vi "Periodic Tasks.vi"(8 "error in":errorcluster) -> ()   [LabVIEW 2014]
doc: "This VI runs in parallel to other tasks. It can contain as many user-defined periodic loops as you need. These can carry out PID or other sorts of timed response."
uses:
  <vilib>/Rock Robotics/WPI/Joystick/WPI_JoystickGetSetRefNum.vi
  <vilib>/Rock Robotics/WPI/RobotDrive/WPI_RobotDriveGetSetRefNum.vi
  <vilib>/Rock Robotics/WPI/RobotDrive/WPI_RobotDriveMotorSelectorEnum.ctl
  <vilib>/Rock Robotics/SystemInterfaces/NetworkCommunication/NetComm_UsageReport_ResourceType.ctl
  <vilib>/addons/control/pid/NI_PID_pid.lvlib
  <vilib>/addons/control/pid/pid.llb/PID (DBL).vi
  Robot Global Data.vi
  robotics/labview/nav6/roborio/labview/Nav6Library/Nav6.lvlib
panel:
  out "Motor Values":dbl[](array[numeric])
  in  "Gyro Angle":dbl
  in  "error in (no error)":errorcluster
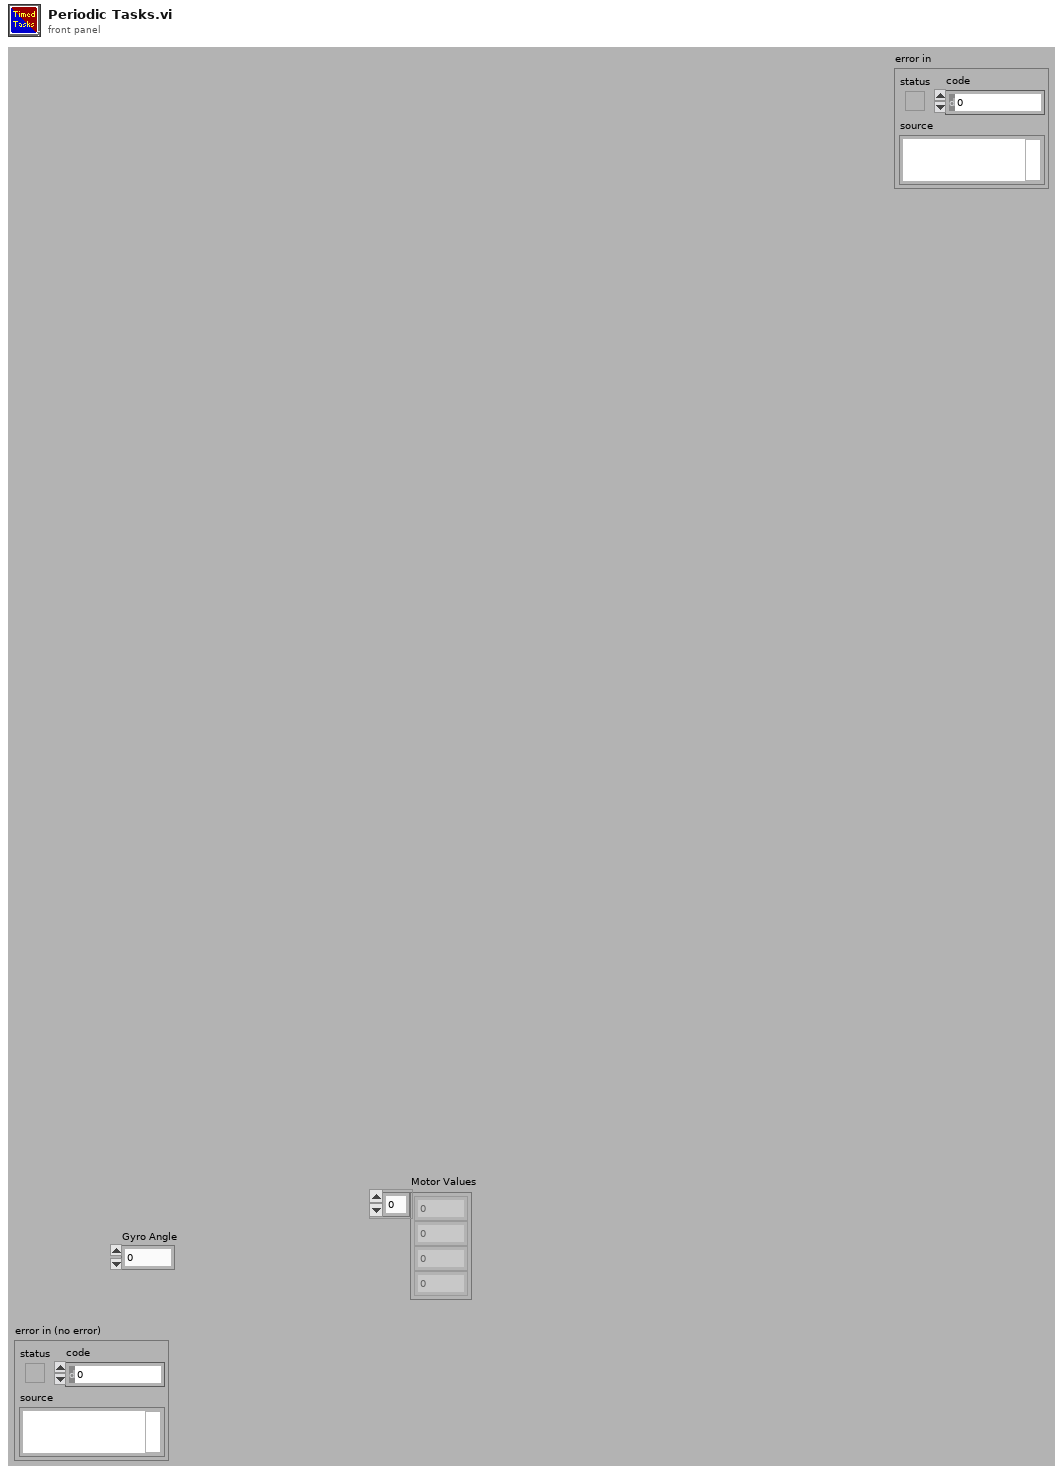
[diagram p1: front panel]
types:
  T1 = typedef "NetComm_UsageReport_ResourceType.ctl" = enum8{"Controller", "Module", "Language", "CANPlugin", "Accelerometer", "ADXL345", "AnalogChannel", "AnalogTrigger", "AnalogTriggerOutput", "CANJaguar", "Compressor", "Counter", "Dashboard", "DigitalInput", "DigitalOutput", "DriverStationCIO", "DriverStationEIO", "DriverStationLCD", "Encoder", "GearTooth", "Gyro", "I2C", "Framework", "Jaguar", "Joystick", "Kinect", "KinectStick", "PIDController", "Preferences", "PWM", "Relay", "RobotDrive", "SerialPort", "Servo", "Solenoid", "SPI", "Task", "Ultrasonic", "Victor", "Button", "Command", "AxisCamera", "PCVideoServer", "SmartDashboard", "Talon", "HiTechnicColorSensor", "HiTechnicAccel", "HiTechnicCompass", "SRF08", "AnalogOutput", "Victor SP", "Talon SRX", "CAN Talon SRX"}
  T2 = typedef "WPI_RobotDriveMotorSelectorEnum.ctl" = enum16{"Rear Left Motor", "Rear Right Motor", "Front Left Motor", "Front Right Motor"}
  T3 = typedef "WPI_DriverStationRobotMode2.ctl" = enum16{"Autonomous Disabled", "Autonomous Enabled", "Teleop Disabled", "Teleop Enabled", "Disconnected", "Finish", "Test Disabled", "Test Enabled", "Emergency Stopped"}
  T4 = typedef "WPI_JoystickDevRef.ctl" = cluster{"Device":T5}
  T5 = typedef "WPI_JoystickDeviceEnum.ctl" = enum16{"USB 0", "USB 1", "USB 2", "USB 3", "USB 4", "USB 5"}
  T6 = typedef "WPI_RobotDriveDevRef.ctl" = cluster{"DevStatus":errorcluster, "Motors[]":T7[], "Square Inputs":bool, "Max Output":dbl}
  T7 = typedef "WPI_MotorControlDeviceRef.ctl" = cluster{"DeviceStatus":errorcluster, "Type":T8, "PWM":cluster{"Controller":T9, "PWM Channel":T10, "DeadBand":T11}, "CAN":cluster{"Device Number":u8, "Control Mode":T12, "Semaphore":T13, "Max Vout":dbl, "TalonSRX Control Mode":T14}, "Invert":bool, "TransformRef":T15, "InvTransformRef":T15}
  T8 = typedef "WPI_MotorControlType.ctl" = enum16{"PWM", "CAN", "CANTalonSRX"}
  T9 = typedef "FPGA_TypedefDigitalModule.ctl" = enum16{"Controller 1"}
  T10 = typedef "FPGA_DIOPWMChannel.ctl" = enum8{"PWM 0", "PWM 1", "PWM 2", "PWM 3", "PWM 4", "PWM 5", "PWM 6", "PWM 7", "PWM 8", "PWM 9", "PWM MXP 0", "PWM MXP 1", "PWM MXP 2", "PWM MXP 3", "PWM MXP 4", "PWM MXP 5", "PWM MXP 6", "PWM MXP 7", "PWM MXP 8", "PWM MXP 9", "Invalid"}
  T11 = typedef "WPI_PWMDeadband.ctl" = cluster{"Name":string, "maxPositivePwm":i32, "minPositivePwm":i32, "centerPwm":i32, "maxNegativePwm":i32, "minNegativePwm":i32, "angularRange":u16}
  T12 = typedef "WPI_CANJaguar_ControlMode.ctl" = enum8{"Percent VBus", "Current", "Speed", "Position", "Voltage"}
  T13 = typedef "Semaphore RefNum" = refnum<k1>
  T14 = typedef "WPI_CANTalonSRX_APIControlMode.ctl" = enum8{"Percent VBus", "Speed", "Position", "Slave", "Unchanged / Invalid"}
  T15 = typedef "WPI_PWMTransform_ConPane.ctl" = refnum<vi>
  T16 = cluster{"proportional gain (Kc)":dbl, "integral time (Ti, min)":dbl, "derivative time (Td, min)":dbl}
  T17 = cluster{"JoystickDevRef":T4, "RobotDriveDevRef":T6}
  T18 = typedef "Nav6.lvlib/Nav6DevRef.ctl" = cluster{"SerialPortRef":T19, "UpdateRate":u8, "Error":errorcluster, "Nav6Mode":T20}
  T19 = typedef "WPI_SerialPortRef.ctl" = cluster{"DevStatus":errorcluster, "Serial Port Name":refnum<visa-resource-name>}
  T20 = typedef "Nav6.lvlib/Nav6Mode.ctl" = enum16{"YPR", "Gyro", "Quaternion"}
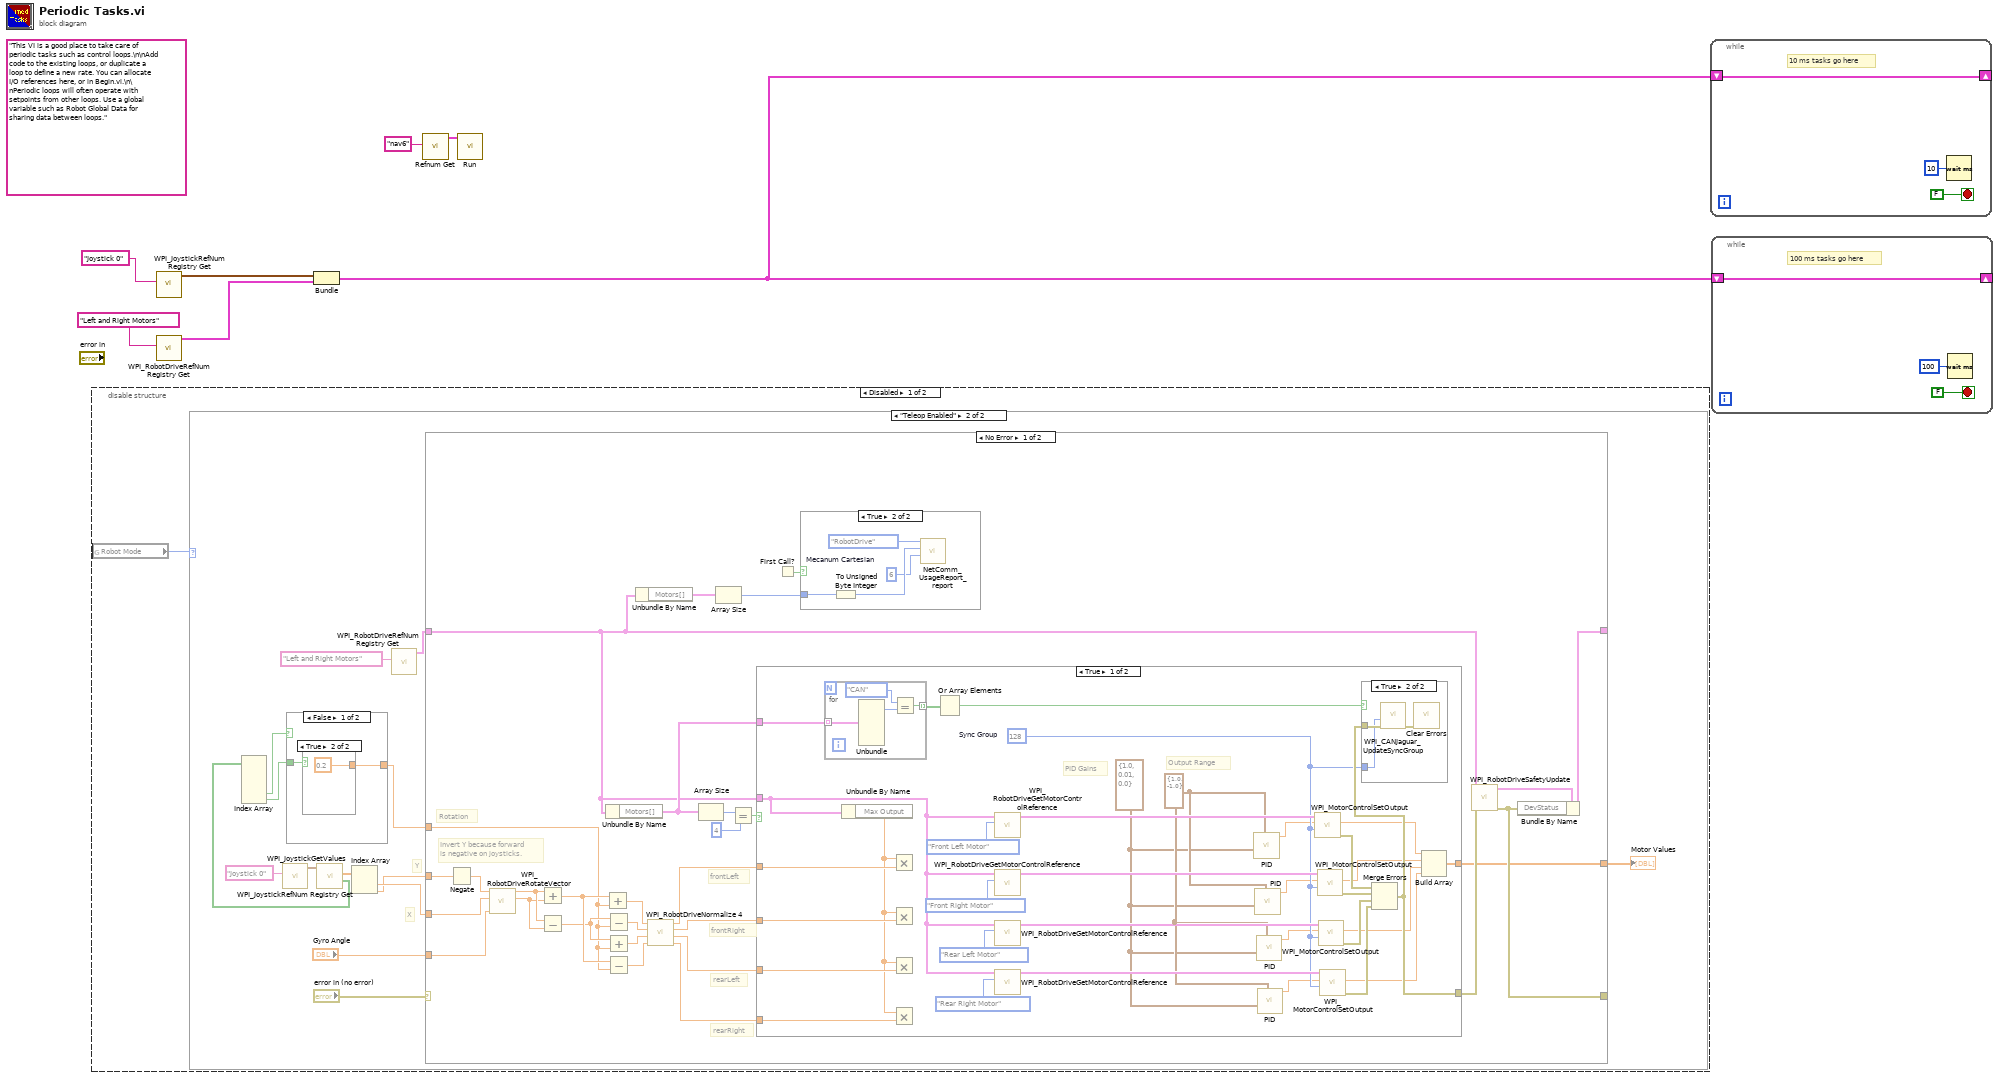
[diagram p0: block diagram]
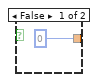
[diagram p3: hidden frame]
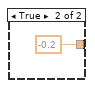
[diagram p4: hidden frame]
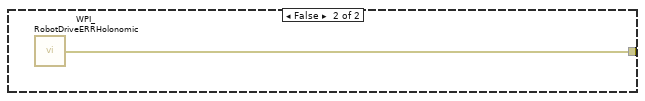
[diagram p7: hidden frame]
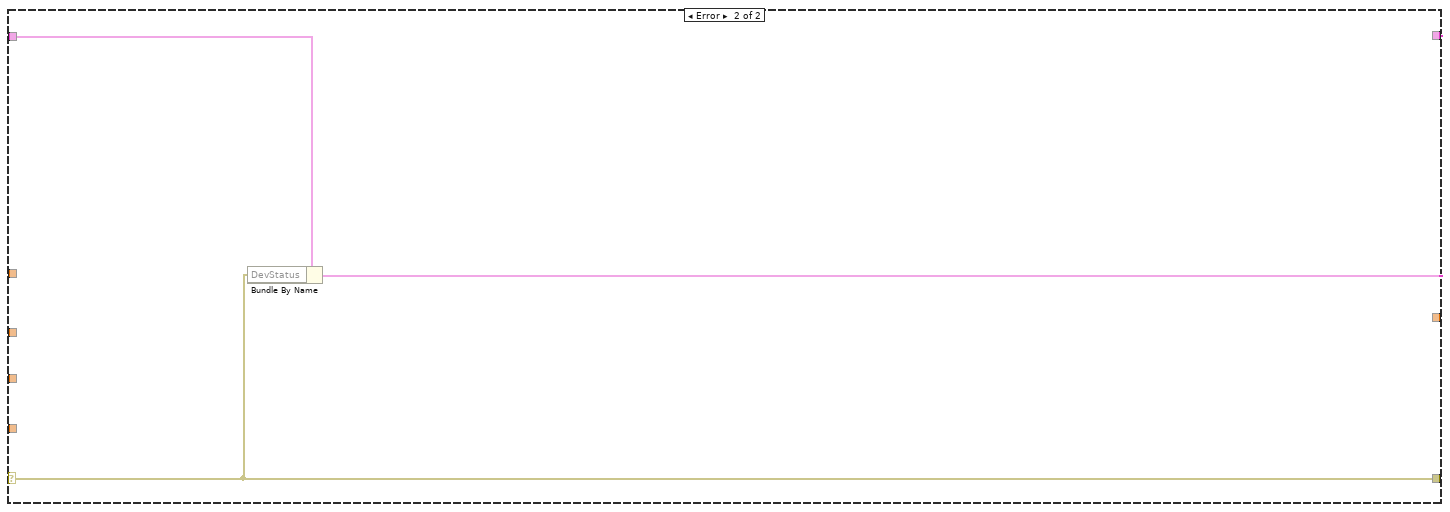
[diagram p8: hidden frame]
diagram:
  (unwired) "This VI is a good place to take care of periodic tasks such as control loops.\n\nAdd code to the existing loops, or duplicate a loop to define a new rate. You can allocate I/O references here, or in Begin.vi.\n\nPeriodic loops will often operate with setpoints from other loops. Use a global variable such as Robot Global Data for sharing data between loops."
  n1 = disable-structure shown="Disabled" {
    frame Disabled {
      n2 = global read "Robot Global Data.vi" "Robot Mode"() -> (w8:T3)
      n3 = case shown="\"Teleop Enabled\"" w8 {
        frame "Teleop Disabled", Default {
        }
        frame "Teleop Enabled" {
          # "X"
          # "Y"
          n4 = call <vilib>:"WPI_JoystickRefNum Registry Get.vi"("refnum name"="Joystick 0") -> ("JoystickDevRef"=w16:T4)  [unwired: 1 in, 9 out]
          n5 = call <vilib>:"WPI_JoystickGetValues.vi"("JoystickDevRef"=w16) -> ("Buttons"=w9:bool[], "Axes"=w15:dbl[])  [unwired: 6 in, 3 out]
          n6 = Index Array(array=w9) -> (element #4=w11:bool, element #5=w10:bool)  [unwired: 5 in, 3 out]
          n7 = case shown="False" w11 {
            tunnel: w10 -> [w24 _]
            tunnel: [w23 -0.2] -> w12
            frame False {
              n8 = case shown="True" w24 {
                tunnel: [0 0.2] -> w23
                frame False {
                }
                frame True {
                }
              }
            }
            frame True {
            }
          }
          n9 = Index Array(array=w15) -> (element #1=w14:dbl, element #2=w13:dbl)  [unwired: 2 in]
          n10 = call <vilib>:"WPI_RobotDriveRefNum Registry Get.vi"("refnum name"="Left and Right Motors") -> ("RobotDriveDevRef"=w19:T6)  [unwired: 1 in, 9 out]
          n11 = case shown="No Error" "error in (no error)" {
            selector: "error in (no error)" -> [_ w104]
            tunnel: w13 -> [w39 _]
            tunnel: w14 -> [w44 _]
            tunnel: w19 -> [w29 w106]
            tunnel: [w54 w105] -> _
            tunnel: [w34 w104] -> _
            tunnel: w12 -> [w45 _]
            tunnel: "Gyro Angle" -> [w38 _]
            tunnel: [w28 _] -> w20
            frame No Error {
              # "Rotation"
              # "Invert Y because forward is negative on joysticks."
              # "rearLeft"
              # "frontRight"
              # "rearRight"
              # "frontLeft"
              n12 = Negate(x=w39) -> (-x=w37:dbl)
              n13 = call <vilib>:"WPI_RobotDriveRotateVector.vi"("Angle"=w38, "X"=w44, "Y"=w37) -> ("X'"=w52:dbl, "Y'"=w53:dbl)  [unwired: 7 out]
              n14 = Add(x=w53, y=w52) -> (x+y=w50:dbl)
              n15 = Subtract(x=w53, y=w52) -> (x-y=w48:dbl)
              n16 = Add(x=w50, y=w45) -> (x+y=w46:dbl)
              n17 = Unbundle By Name(w29) -> ("Motors[]"=w33:T7[])
              n18 = Subtract(x=w48, y=w45) -> (x-y=w47:dbl)
              n19 = Add(x=w48, y=w45) -> (x+y=w49:dbl)
              n20 = Subtract(x=w50, y=w45) -> (x-y=w51:dbl)
              n21 = Unbundle By Name(w29) -> ("Motors[]"=w31:T7[])
              n22 = call <vilib>:"WPI_RobotDriveNormalize 4.vi"("D"=w51, "C"=w49, "B"=w47, "A"=w46) -> ("D'"=w41:dbl, "C'"=w40:dbl, "B'"=w42:dbl, "A'"=w43:dbl)
              n23 = Array Size(array=w33) -> (size(s)=w57:i32)
              n24 = Array Size(array=w31) -> (size(s)=w30:i32)
              n25 = Equal?(x=w57, y=4) -> (x = y?=w55:bool)
              n26 = case shown="True" w55 {
                tunnel: w43 -> [w95 _]
                tunnel: w42 -> [w94 _]
                tunnel: w29 -> [w83 _]
                tunnel: [w74 w103] -> w36
                tunnel: w40 -> [w89 _]
                tunnel: w41 -> [w88 _]
                tunnel: w33 -> [w75 _]
                tunnel: [w71 _] -> w28
                frame True {
                  w62 = T16 {"proportional gain (Kc)"=1.0, "integral time (Ti, min)"=0.01, "derivative time (Td, min)"=0.0} ("PID gains")
                  w63 = cluster{"output high":dbl, "output low":dbl} {"output high"=1.0, "output low"=-1.0} ("output range")
                  w73 = u8 128  # Sync Group
                  # "Output Range"
                  # "PID Gains"
                  n27 = for {
                    tunnel: w75 -> [w99] mode=indexing
                    tunnel: [w96] -> w76 mode=indexing
                    n28 = Unbundle(w99) -> ("Type"=w98:T8)  [unwired: 6 out]
                    n29 = Equal?(x=enum16{"PWM", "CAN"}."CAN" ("Type"), y=w98) -> (x = y?=w96:bool)
                  }
                  n30 = Unbundle By Name(w83) -> ("Max Output"=w82:dbl)
                  n31 = Multiply(x=w82, y=w95) -> ()  [unwired: 1 out]
                  n32 = Multiply(x=w82, y=w94) -> ()  [unwired: 1 out]
                  n33 = Multiply(x=w82, y=w89) -> ()  [unwired: 1 out]
                  n34 = Multiply(x=w82, y=w88) -> ()  [unwired: 1 out]
                  n35 = Or Array Elements(Boolean array=w76) -> (logical OR=w77:bool)
                  n36 = call <vilib>:"WPI_RobotDriveGetMotorControlReference.vi"("MotorIndex"=WPI_RobotDriveMotorSelectorEnum."Front Left Motor", "RobotDriveDevRef"=w83) -> ("MotorControlDeviceRef"=w93:T7)  [unwired: 9 out]
                  n37 = call <vilib>:"WPI_RobotDriveGetMotorControlReference.vi"("MotorIndex"=WPI_RobotDriveMotorSelectorEnum."Front Right Motor", "RobotDriveDevRef"=w83) -> ("MotorControlDeviceRef"=w91:T7)  [unwired: 9 out]
                  n38 = call <vilib>:"WPI_RobotDriveGetMotorControlReference.vi"("MotorIndex"=WPI_RobotDriveMotorSelectorEnum."Rear Left Motor", "RobotDriveDevRef"=w83) -> ("MotorControlDeviceRef"=w92:T7)  [unwired: 9 out]
                  n39 = call <vilib>:"WPI_RobotDriveGetMotorControlReference.vi"("MotorIndex"=WPI_RobotDriveMotorSelectorEnum."Rear Right Motor", "RobotDriveDevRef"=w83) -> ("MotorControlDeviceRef"=w90:T7)  [unwired: 9 out]
                  n40 = call-poly <vilib>:"PID.vi"("output range"=w63, "PID gains"=w62) -> ("output"=w66:dbl)  [unwired: 8 in, 1 out]
                  n41 = call-poly <vilib>:"PID.vi"("output range"=w63, "PID gains"=w62) -> ("output"=w65:dbl)  [unwired: 8 in, 1 out]
                  n42 = call-poly <vilib>:"PID.vi"("output range"=w63, "PID gains"=w62) -> ("output"=w64:dbl)  [unwired: 8 in, 1 out]
                  n43 = call-poly <vilib>:"PID.vi"("output range"=w63, "PID gains"=w62) -> ("output"=w67:dbl)  [unwired: 8 in, 1 out]
                  n44 = call <vilib>:"WPI_MotorControlSetOutput.vi"("Sync Group / Parameter Slot"=w73, "Output"=w66, "MotorControlDevRef"=w93) -> ("error out"=w78:errorcluster, "Motor Output"=w72:dbl)  [unwired: 2 in, 5 out]
                  n45 = call <vilib>:"WPI_MotorControlSetOutput.vi"("Sync Group / Parameter Slot"=w73, "Output"=w65, "MotorControlDevRef"=w91) -> ("error out"=w79:errorcluster, "Motor Output"=w70:dbl)  [unwired: 2 in, 5 out]
                  n46 = call <vilib>:"WPI_MotorControlSetOutput.vi"("Sync Group / Parameter Slot"=w73, "Output"=w64, "MotorControlDevRef"=w92) -> ("error out"=w80:errorcluster, "Motor Output"=w69:dbl)  [unwired: 2 in, 5 out]
                  n47 = call <vilib>:"WPI_MotorControlSetOutput.vi"("Sync Group / Parameter Slot"=w73, "Output"=w67, "MotorControlDevRef"=w90) -> ("error out"=w81:errorcluster, "Motor Output"=w68:dbl)  [unwired: 2 in, 5 out]
                  n48 = Merge Errors(w78, w79, w80, w81) -> (w74:errorcluster)
                  n49 = case shown="True" w77 {
                    tunnel: w74 -> [_ w101]
                    tunnel: w73 -> [_ w100]
                    frame False {
                    }
                    frame True {
                      n50 = call <vilib>:"WPI_CANJaguar_UpdateSyncGroup.vi"("error in (no error)"=w101, "Sync Group"=w100) -> ("error out"=w102:errorcluster)  [unwired: 9 out]
                      n51 = call <vilib>:"Clear Errors.vi"("error in (no error)"=w102) -> ()  [unwired: 1 in, 6 out]
                    }
                  }
                  n52 = Build Array(w72, w70, w69, w68) -> (w71:dbl[])
                }
                frame False {
                  n53 = call <vilib>:"WPI_RobotDriveERRHolonomic.vi"() -> ("error out"=w103:errorcluster)
                }
              }
              n54 = First Call?() -> (First Call?: T/F=w32:bool)
              n55 = case shown="True" w32 {
                tunnel: w30 -> [_ w60]
                frame False {
                }
                frame True {
                  w58 = u8 6  # Mecanum Cartesian
                  n56 = To Unsigned Byte Integer(number=w60) -> (unsigned 8bit integer=w59:u8)
                  n57 = call <vilib>:"NetComm_UsageReport_report.vi"("Context"=w58, "Instance Number"=w59, "Resource Type"=NetComm_UsageReport_ResourceType."RobotDrive") -> ()  [unwired: 9 in]
                }
              }
              n58 = call <vilib>:"WPI_RobotDriveSafetyUpdate.vi"("error in (no error)"=w36, "RobotDriveDevRef"=w29) -> ("error out"=w34:errorcluster, "RobotDriveDevRef"=w35:T6)  [unwired: 8 out]
              n59 = Bundle By Name(cluster=w35, "DevStatus"=w34) -> (w54:T6)
            }
            frame Error {
              n60 = Bundle By Name(cluster=w106, "DevStatus"=w104) -> (w105:T6)
            }
          }
          "Motor Values" <- w20
        }
      }
    }
    frame Enabled {
    }
  }
  n61 = call <vilib>:"WPI_JoystickRefNum Registry Get.vi"("refnum name"="Joystick 0") -> ("JoystickDevRef"=w5:T4)  [unwired: 1 in, 9 out]
  n62 = call <vilib>:"WPI_RobotDriveRefNum Registry Get.vi"("refnum name"="Left and Right Motors") -> ("RobotDriveDevRef"=w4:T6)  [unwired: 1 in, 9 out]
  n63 = Bundle("JoystickDevRef"=w5, "RobotDriveDevRef"=w4) -> (w3:T17)  [unwired: 1 out]
  n64 = call "Refnum Get.vi"("refnum name"="nav6") -> ("Nav6DevRef"=w2:T18)  [unwired: 9 in, 1 out]
  n65 = call "Run.vi"("Nav6DevRef"=w2) -> ()  [unwired: 11 in]
  n66 = while {
    shift-right: [w107] -> _
    shift-left: w3 -> [w107]
    stop <- FALSE stop-if-true
    # "10 ms tasks go here"
    n67 = Wait (ms)(milliseconds to wait=u32 10) -> ()  [unwired: 1 out]
  }
  n68 = while {
    shift-right: [w110] -> _
    shift-left: w3 -> [w110]
    stop <- FALSE stop-if-true
    # "100 ms tasks go here"
    n69 = Wait (ms)(milliseconds to wait=u32 100) -> ()  [unwired: 1 out]
  }
